vi "CRYData & result stacks global.vi"() -> ()   [LabVIEW 2013]
panel:
  in  "Tested # No sum":u16
  in  "Always replace":bool
  in  "Tested #":u16
  in  "Last file offsets":cluster{"path":path, "offset":i32}[](array[cluster])
  in  "Lot #":string="00"
  in  "Serial #":string="00"
  in  "prev Serial #":string="00"
  in  "Redo":bool
  in  "Pause":bool
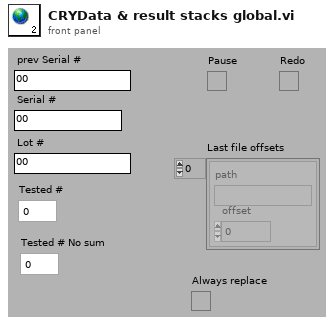
[diagram p1: front panel]
diagram:
